vi "Send Return Events.vi"(7 "Message Priority (Normal)":T1=enum."Normal", 8 "error in (no error)":errorcluster, 10 "Event Reply Queue In":refnum<queue>, 11 "Message Enqueuer":refnum<class "Message Enqueuer.lvclass">) -> (0 "error out":errorcluster, 2 "Event Reply Queue Out":refnum<queue>, 3 "Message Enqueuer out":refnum<class "Message Enqueuer.lvclass">)   [LabVIEW 2015, in "Command Handler.lvlib" / "Return Events Msg.lvclass"]
doc: "This VI sends the message to an actor."
uses:
  Return Events Msg.lvclass
  <vilib>/ActorFramework/Message Enqueuer/Message Enqueuer.lvclass
  <vilib>/ActorFramework/Message Enqueuer/Message Priority.ctl
  Command Handler/Type Defs/Event Cluster.ctl
  Command Handler/Command Handler.lvclass
  Command Handler/Type Defs/Command Handler Data.ctl
  Command Parent/Command.lvclass
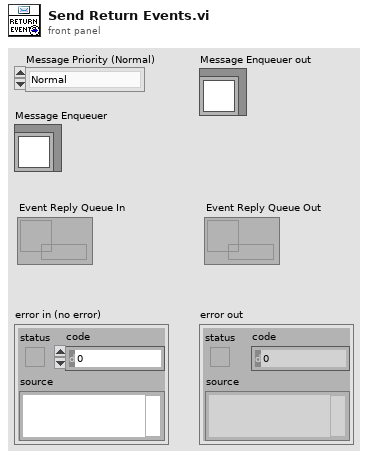
[diagram p1: front panel]
types:
  T1 = typedef "Actor Framework.lvlib/Message Enqueuer.lvclass/Message Priority.ctl" = enum16{"Low", "Normal", "High"}
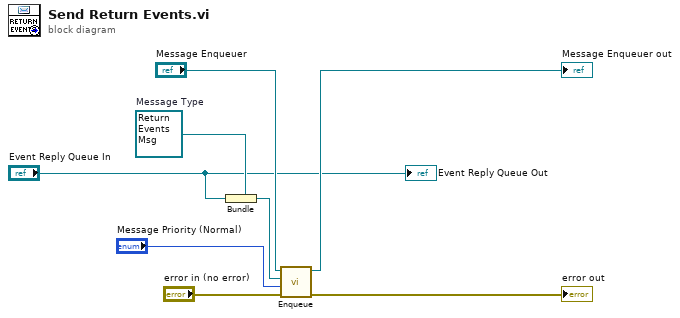
[diagram p0: block diagram]
diagram:
  w6 = refnum<class "Return Events Msg.lvclass"> refnum  # Message Type
  n1 = Bundle(cluster=w6, "Event Reply Queue In") -> (w5:refnum<class "Return Events Msg.lvclass">)
  n2 = call <vilib>:"Enqueue.vi"("error in (no error)"="error in (no error)", "Message Priority (Normal)"="Message Priority (Normal)", "Message"=w5, "Message Enqueuer in"="Message Enqueuer") -> ("error out"=→"error out":errorcluster, "Message Enqueuer out"=→"Message Enqueuer out":refnum<class "Message Enqueuer.lvclass">)  [unwired: 6 in]
  "Event Reply Queue Out" <- "Event Reply Queue In"
